vi "dictionary_processing_test.vi"() -> ()   [LabVIEW 2016]
uses:
  <userlib>/_OpenG.lib/dictionary/dictionary.llb/Dictionary Update (by scalar value)__ogtk.vi
  <userlib>/LevyLab/XY Utilities/subVIs/Derivative (multiple).vi
  <userlib>/LevyLab/XY Utilities/xy_utilities.lvlib
panel:
  in  "xy input":T1(array[cluster])
  out "XY Graph 2":cluster{"Intensity Data":dbl[], "Array":dbl[]}[](graph)
  out "XY Graph":cluster{"Intensity Data":dbl[], "Array":dbl[]}[](graph)
  in  "Array":i32[](array[numeric])=[0, 0]
  in  "derivative":T2={"derivative"="derivative", "Interval"=2.0, "Interval Units"=enum."Points", "Type"=enum."dy/dx vs x"}
  out "xy output":cluster{dbl[], "magnitude":dbl[]}[](array[cluster])
  out "output data":dbl[][](graph)
  in  "input data":dbl[][](graph)
  out "Element Names":string[][](array[string])
  out "Numeric":i32
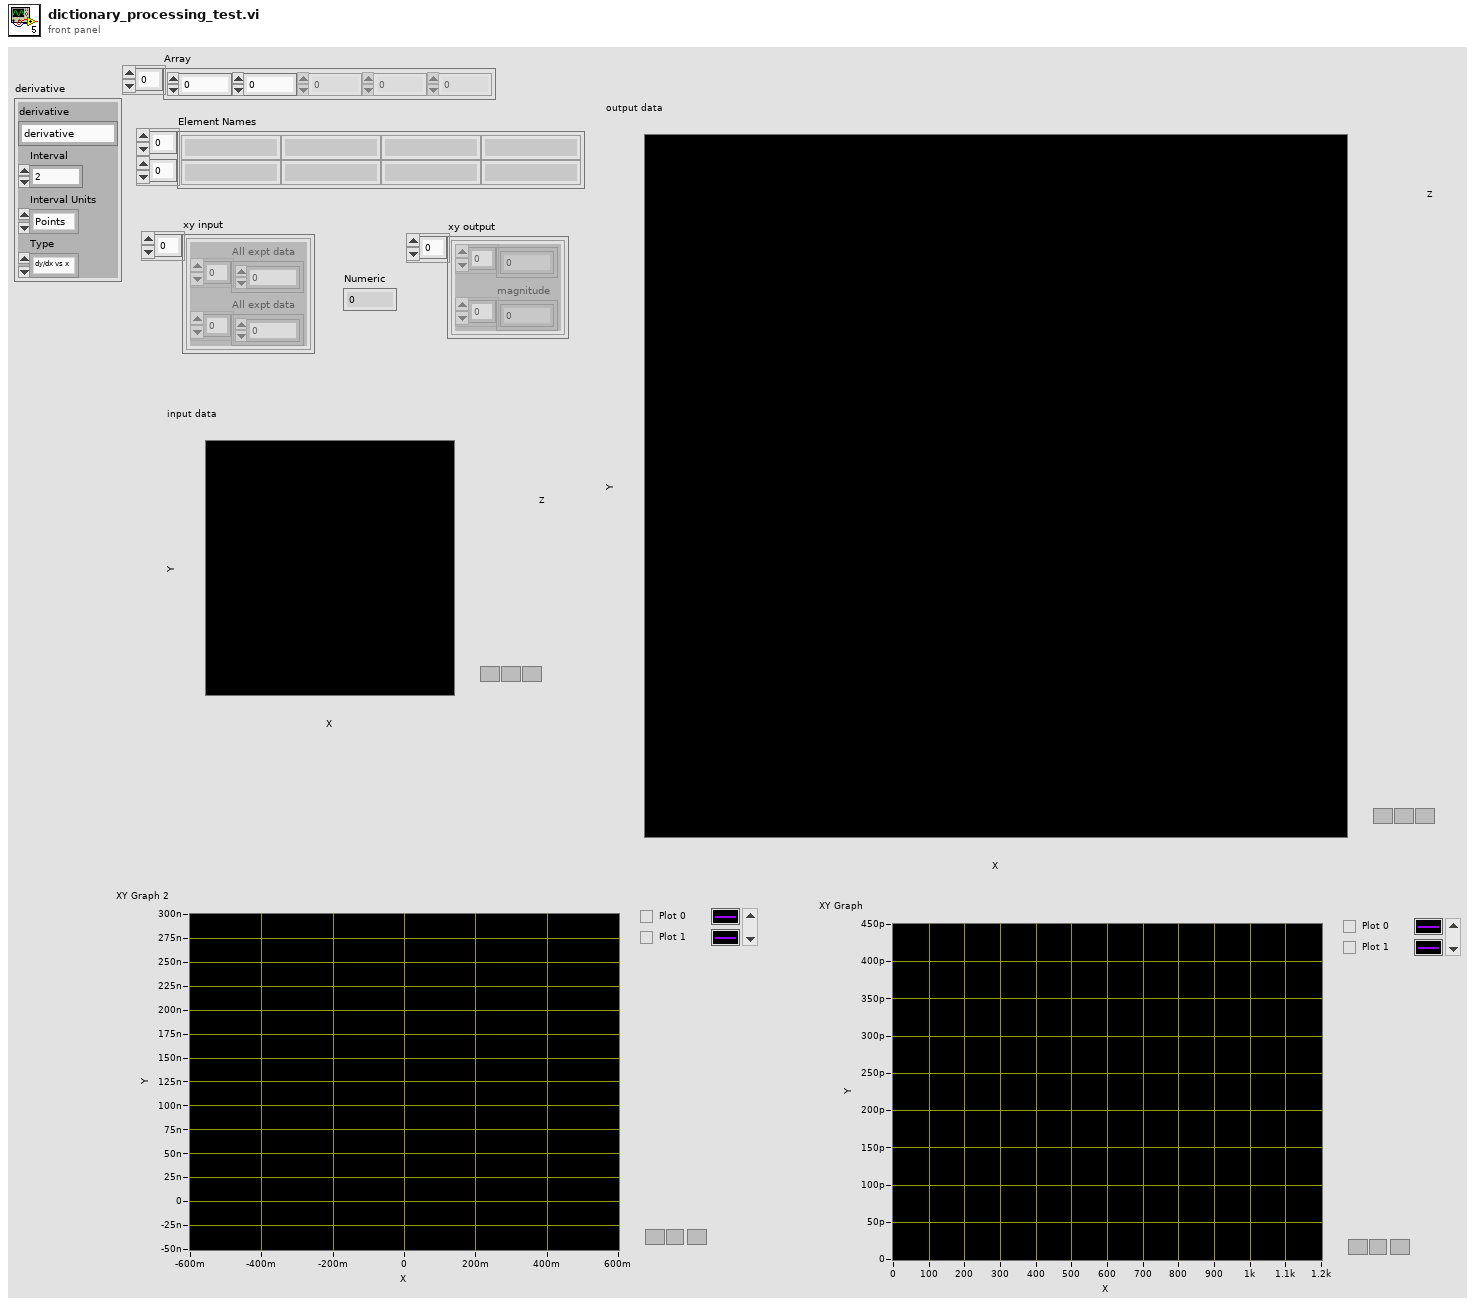
[diagram p1: front panel]
types:
  T1 = cluster{"All expt data":dbl[], "All expt data":dbl[]}[]
  T2 = cluster{"derivative":string, "Interval":dbl, "Interval Units":enum16{"Points", "Data"}, "Type":enum16{"dy/dx vs x", "dx/dy vs y"}}
  T3 = typedef "Dictionary Object RefNum__ogtk.ctl" = refnum<k1>
  T4 = cluster{i32, "derivative":cluster{"derivative":string, "Interval":dbl, "Interval Units":enum16{"Points", "Data"}, "Type":enum16{"dy/dx vs x", "dx/dy vs y"}}}
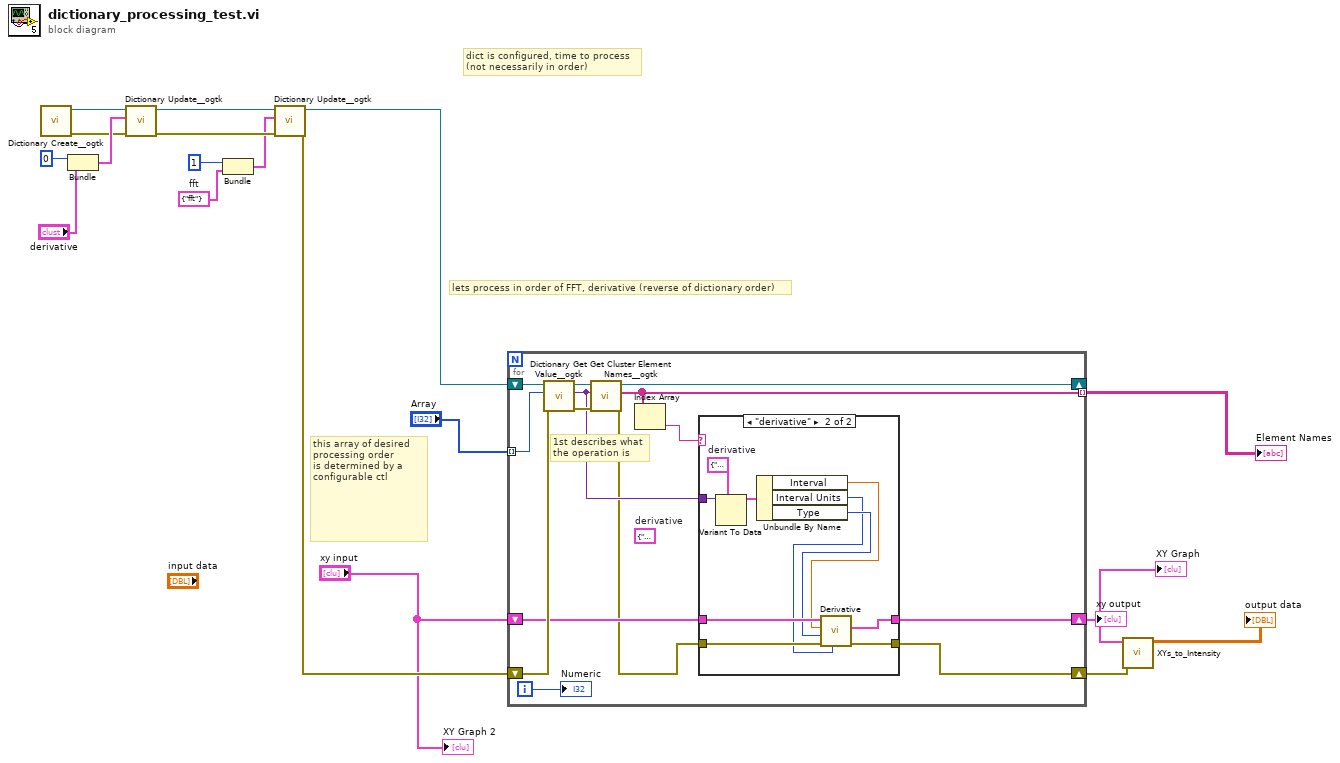
[diagram p0: block diagram]
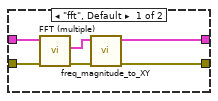
[diagram p2: hidden frame]
diagram:
  w4 = cluster{"fft":string} {"fft"="fft"}  # fft
  # "this array of desired processing order\nis determined by a configurable ctl"
  # "lets process in order of FFT, derivative (reverse of dictionary order)"
  # "dict is configured, time to process\n(not necessarily in order)"
  n1 = call <userlib>:"Dictionary Create__ogtk.vi"() -> ("error out"=w8:errorcluster, "dictionary out"=w18:T3)  [unwired: 10 in]
  n2 = Bundle(0, "derivative"="derivative") -> (w17:T4)  [unwired: 1 in]
  n3 = call-poly <userlib>:"Dictionary Update__ogtk.vi"("error in (no error)"=w8, "key-value"=w17, "dictionary"=w18) -> ("error out"=w9:errorcluster, "dictionary out"=w14:T3)  [unwired: 6 in, 1 out]
  n4 = Bundle(1, "fft"=w4) -> (w3:cluster{i32, "fft":cluster{"fft":string}})  [unwired: 1 in]
  n5 = call-poly <userlib>:"Dictionary Update__ogtk.vi"("error in (no error)"=w9, "key-value"=w3, "dictionary"=w14) -> ("error out"=w10:errorcluster, "dictionary out"=w12:T3)  [unwired: 6 in, 1 out]
  n6 = for {
    tunnel: "Array" -> [w30] mode=indexing
    shift-right: [w29] -> _
    shift-left: w12 -> [w31]
    tunnel: [w27] -> w11 mode=indexing
    shift-right: [w19] -> w6
    shift-left: w10 -> [w24]
    shift-right: [w21] -> w2
    shift-left: "xy input" -> [w22]
    i -> [w28]
    (unwired) T2 {"derivative"="derivative", "Interval"=2.0, "Interval Units"=enum."Points", "Type"=enum."dy/dx vs x"}  # derivative
    # "1st describes what\nthe operation is"
    n7 = call <userlib>:"Dictionary Get Value__ogtk.vi"("error in"=w24, "key"=w30, "dictionary"=w31) -> ("error out"=w25:errorcluster, "value"=w23:variant, "dictionary out"=w29:T3)  [unwired: 5 in, 1 out]
    n8 = call <userlib>:"Get Cluster Element Names__ogtk.vi"("error in (no error)"=w25, "Cluster"=w23) -> ("error out"=w20:errorcluster, "Element Names"=w27:string[])  [unwired: 8 in]
    n9 = Index Array(array=w27) -> (element=w26:string)  [unwired: 1 in]
    n10 = case shown="\"derivative\"" w26 {
      tunnel: w23 -> [_ w46]
      tunnel: w22 -> [w37 w43]
      tunnel: [w33 w42] -> w21
      tunnel: w20 -> [w36 w44]
      tunnel: [w34 w41] -> w19
      frame "fft", Default {
        n11 = call <userlib>:"FFT (multiple).vi"("error in (no error)"=w36, "XY-data"=w37) -> ("error out"=w35:errorcluster, "magnitude []"=w32:cluster{"f0":dbl, "df":dbl, "magnitude":dbl[]}[])  [unwired: 6 in, 2 out]
        n12 = call "freq_magnitude_to_XY.vi"("error in (no error)"=w35, "magnitude []"=w32) -> ("error out"=w34:errorcluster, "freq_magnitude_XY"=w33:cluster{dbl[], "magnitude":dbl[]}[])  [unwired: 8 in]
      }
      frame "derivative" {
        w45 = T2 {"derivative"="derivative", "Interval"=2.0, "Interval Units"=enum."Points", "Type"=enum."dy/dx vs x"}  # derivative
        n13 = Variant To Data(type=w45, Variant=w46) -> (data=w47:T2)  [unwired: 1 in, 1 out]
        n14 = Unbundle By Name(w47) -> ("Interval"=w40:dbl, "Interval Units"=w38:enum16{"Points", "Data"}, "Type"=w39:enum16{"dy/dx vs x", "dx/dy vs y"})
        n15 = call-poly <userlib>:"Derivative.vi"("Interval Units"=w38, "error in (no error)"=w44, "Type"=w39, "Interval"=w40, "XY-data"=w43) -> ("error out"=w41:errorcluster, "Differential out"=w42:cluster{"X-array":dbl[], "Y-array":dbl[]}[])  [unwired: 4 in, 1 out]
      }
    }
    "Numeric" <- w28
  }
  "Element Names" <- w11
  "xy output" <- w2
  "XY Graph" <- w2
  n16 = call "XYs_to_Intensity.vi"("error in (no error)"=w6, "XYs in"=w2) -> ("Intensity data (y) out"=→"output data":dbl[][])  [unwired: 8 in, 1 out]
  "XY Graph 2" <- "xy input"
